vi "get current selections.vi"(8 "error in (no error)":errorcluster, 10 "Meet Filter Requirements (T)":bool=TRUE, 11 "Tree in":refnum<class "alias-tree.lvclass">) -> (0 "error out":errorcluster, 2 "Selected Paths":string[](array[string]), 3 "Tree out":refnum<class "alias-tree.lvclass">)   [LabVIEW 2017, in "vs-tree-utility.lvlib" / "alias-tree.lvclass"]
uses:
  alias-tree.lvclass
  NationalInstruments.VeriStand.SystemStorageUI
  NationalInstruments.VeriStand.SystemStorage
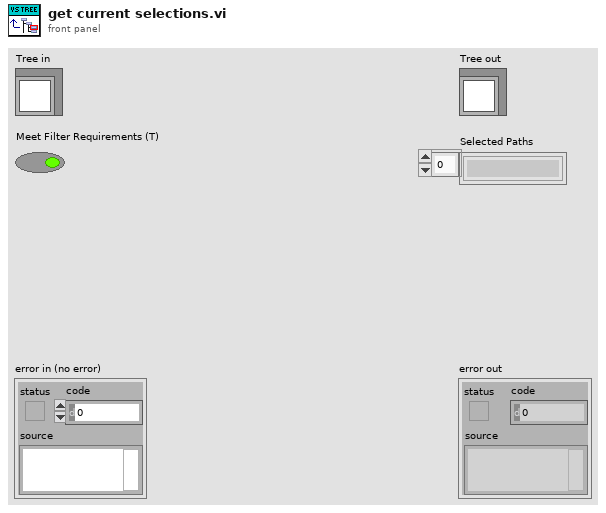
[diagram p1: front panel]
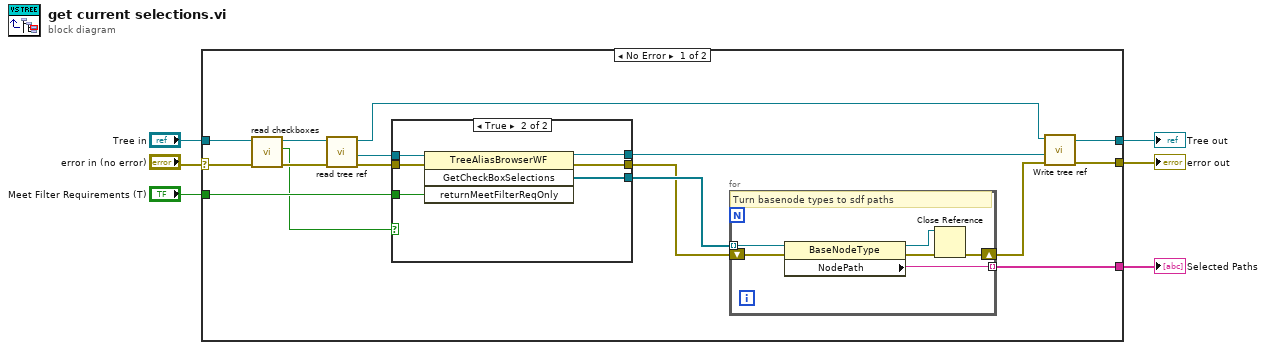
[diagram p0: block diagram]
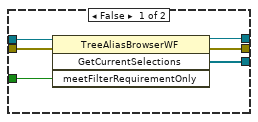
[diagram p2: hidden frame]
diagram:
  n1 = case shown="No Error" "error in (no error)" {
    selector: "error in (no error)" -> [w22 w41]
    tunnel: "Meet Filter Requirements (T)" -> [w21 _]
    tunnel: "Tree in" -> [w10 w42]
    tunnel: [w18 w41] -> w3
    tunnel: [w17 w42] -> w2
    tunnel: [w16 _] -> w1
    frame No Error {
      n2 = call-dynamic "read checkboxes.vi"("error in (no error)"=w22, "alias-tree in"=w10) -> ("error out"=w11:errorcluster, "checkboxes"=w8:bool, "alias-tree out"=w9:refnum<class "alias-tree.lvclass">)  [unwired: 7 in]
      n3 = call-dynamic "read tree ref.vi"("error in (no error)"=w11, "alias-tree in"=w9) -> ("error out"=w20:errorcluster, "tree ref"=w19:refnum<k24>, "alias-tree out"=w7:refnum<class "alias-tree.lvclass">)  [unwired: 7 in]
      n4 = case shown="True" w8 {
        tunnel: w21 -> [w26 w34]
        tunnel: w20 -> [w28 w33]
        tunnel: w19 -> [w27 w32]
        tunnel: [w23 w31] -> w15
        tunnel: [w25 w30] -> w14
        tunnel: [w24 w29] -> w12
        frame False {
          n5 = invoke class="TreeAliasBrowserWF" method="GetCurrentSelections"(reference=w27, error in=w28, "meetFilterRequirementOnly"=w26) -> (reference out=w24:refnum<k24>, error out=w25:errorcluster, "GetCurrentSelections"=w23:refnum<k24>[])  [unwired: 1 in, 1 out]
        }
        frame True {
          n6 = invoke class="TreeAliasBrowserWF" method="GetCheckBoxSelections"(reference=w32, error in=w33, "returnMeetFilterReqOnly"=w34) -> (reference out=w29:refnum<k24>, error out=w30:errorcluster, "GetCheckBoxSelections"=w31:refnum<k24>[])  [unwired: 1 in, 1 out]
        }
      }
      n7 = for {
        tunnel: w15 -> [w40] mode=indexing
        tunnel: [w39] -> w16 mode=indexing
        shift-right: [w36] -> w13
        shift-left: w14 -> [w38]
        # "Turn basenode types to sdf paths"
        n8 = property class="BaseNodeType"(reference=w40, error in=w38) -> (reference out=w35:refnum<k24>, error out=w37:errorcluster, "NodePath"=w39:string)
        n9 = Close Reference(reference=w35, error in (no error)=w37) -> (error out=w36:errorcluster)
      }
      n10 = call-dynamic "Write tree ref.vi"("error in (no error)"=w13, "tree ref"=w12, "alias-tree in"=w7) -> ("error out"=w18:errorcluster, "alias-tree out"=w17:refnum<class "alias-tree.lvclass">)  [unwired: 7 in]
    }
    frame Error {
    }
  }
  "error out" <- w3
  "Tree out" <- w2
  "Selected Paths" <- w1
